vi "Power Output Default Test Parameters.vi"() -> (0 "Default Power Output Test Parameters":T1={"Stimulus"={"Frequency Type"=enum."Band Edges", "Frequency Ranges"=[], "TX 1 Frequency (MHz)"={"Min"=0.0, "Max"=0.0}, "TX 2 Frequency (MHz)"={"Min"=0.0, "Max"=0.0}, "RX Frequency (MHz)"={"Min"=0.0, "Max"=0.0}, "Pad Model Number"="", "Pad Serial Number"="", "Pad Values"=[]}, "Measurement"={"DUT Port"=enum."Port 1", "Direction"=0, "Frequency Step Size"=0}, "Display"={"Frequency"={"Min"=-1.0, "Max"=-1.0}, "Power"={"Min"=-1, "Max"=-1}}, "Limit"={"Min Power (dBm)"=44.0}, "Calibration"={"Calibrated?"=FALSE}} {"Measurement"."Frequency Step Size" items=["0.2", "0.4", "1.0", "2.0", "4.0"]; "Measurement"."Direction" items=["Reverse", "Forward", "Auxiliary"]})   [LabVIEW 2011]
uses:
  TypeDefs/Power Output Test Parameters.ctl
  TypeDefs/Power Output Stimulus Parameters.ctl
  TypeDefs/Power Output Measurement Parameters.ctl
  BPIMCore EXT/HW IO/DUTport.ctl
  BPIMCore EXT/HW IO/MeasMode.ctl
  BPIMCore EXT/HW IO/PIM Sweep Step Size.ctl
  TypeDefs/Power Output Display Parameters.ctl
  TypeDefs/Power Output Limit Parameters.ctl
  TypeDefs/Power Output Calibration State.ctl
panel:
  in  "Saved Power Output Defaults":T1={"Stimulus"={"Frequency Type"=enum."Band Edges", "Frequency Ranges"=[], "TX 1 Frequency (MHz)"={"Min"=0.0, "Max"=0.0}, "TX 2 Frequency (MHz)"={"Min"=0.0, "Max"=0.0}, "RX Frequency (MHz)"={"Min"=0.0, "Max"=0.0}, "Pad Model Number"="", "Pad Serial Number"="", "Pad Values"=[]}, "Measurement"={"DUT Port"=enum."Port 1", "Direction"=0, "Frequency Step Size"=0}, "Display"={"Frequency"={"Min"=-1.0, "Max"=-1.0}, "Power"={"Min"=-1, "Max"=-1}}, "Limit"={"Min Power (dBm)"=44.0}, "Calibration"={"Calibrated?"=FALSE}} {"Measurement"."Frequency Step Size" items=["0.2", "0.4", "1.0", "2.0", "4.0"]; "Measurement"."Direction" items=["Reverse", "Forward", "Auxiliary"]}
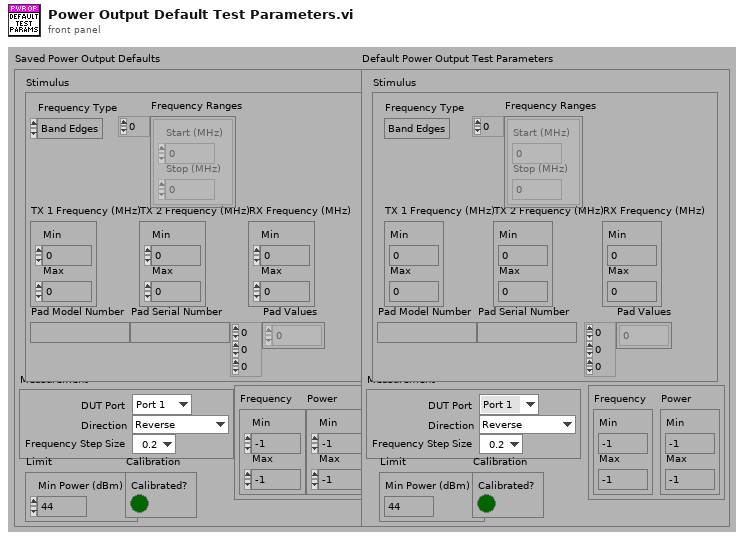
[diagram p1: front panel]
types:
  T1 = typedef "Power Output Test Parameters.ctl" = cluster{"Stimulus":T2, "Measurement":T3, "Display":T7, "Limit":T8, "Calibration":T9}
  T2 = typedef "Power Output Stimulus Parameters.ctl" = cluster{"Frequency Type":enum16{"Band Edges", "Custom"}, "Frequency Ranges":cluster{"Start (MHz)":dbl, "Stop (MHz)":dbl}[], "TX 1 Frequency (MHz)":cluster{"Min":dbl, "Max":dbl}, "TX 2 Frequency (MHz)":cluster{"Min":dbl, "Max":dbl}, "RX Frequency (MHz)":cluster{"Min":dbl, "Max":dbl}, "Pad Model Number":string, "Pad Serial Number":string, "Pad Values":dbl[][][]}
  T3 = typedef "Power Output Measurement Parameters.ctl" = cluster{"DUT Port":T4, "Direction":T5, "Frequency Step Size":T6}
  T4 = typedef "DUTport.ctl" = enum16{"Port 1", "Port 2"}
  T5 = typedef "MeasMode.ctl" = u16
  T6 = typedef "PIM Sweep Step Size.ctl" = u16
  T7 = typedef "Power Output Display Parameters.ctl" = cluster{"Frequency":cluster{"Min":dbl, "Max":dbl}, "Power":cluster{"Min":i32, "Max":i32}}
  T8 = typedef "Power Output Limit Parameters.ctl" = cluster{"Min Power (dBm)":dbl}
  T9 = typedef "Power Output Calibration State.ctl" = cluster{"Calibrated?":bool}
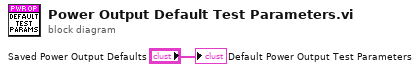
[diagram p0: block diagram]
diagram:
  "Default Power Output Test Parameters" <- "Saved Power Output Defaults"
